vi "Test Cases - API String Arguments Support(VIM).vi"() -> ()   [LabVIEW 2017]
uses:
  2cad2108-17ff-40c4-9c59-29e42dc34fa8.vi
  231c1589-fa39-469a-ad8c-c9d32191fb4b.vi
  479a6c8c-1bad-4955-8cb5-323525784106.vi
  765d0006-b549-469b-b212-20061b8f9c1c.vi
  f8b4bf0f-4264-4187-acce-03e1cac2871a.vi
  390a4868-a891-46e3-9b2d-5b6d63a8fc62.vi
  999417b7-6b4c-4b35-b299-f97fc88c48ae.vi
  e19d2a81-0814-4900-868e-35c1a41a190a.vi
  f192a86a-4283-420b-8c99-03ad7a20a184.vi
  e1086961-258c-488b-92a6-4c27b59b2923.vi
  68628d2e-6ea5-433a-a027-c32794422804.vi
  23749281-1039-457a-b950-e2c2784c1fed.vi
  79993085-fdde-4ff4-95ba-e023c3552d6a.vi
  API-String-Arugments-Support/_Support/Convert API String Arguments to Data(variant).vi
panel:
  out "Cluster":cluster{"2d":dbl[][]}={"2d"=[[3.12, 4.113, 2.3, 5.0, 5.0, 2.3, 4.11, 5.0]]}
  in  "String 13":string="[3.12,4.113,2.3,5;3.12,5,2.3;3.12,4.11,5]"
  out "error 13":errorcluster
  in  "String 12":string="[3.12,4.113,2.3,5;3.12,5,2.3;3.12,4.11,5]"
  out "error 12":errorcluster
  out "Data 11":dbl[][](array[numeric])=[[3.12, 4.113, 2.3, 5.0, 5.0, 2.3, 4.11, 5.0]]
  in  "String 11":string="[{Bool:Off;child.name:ddd},{Bool:On;name:ddd}]"
  out "error 11":errorcluster
  out "Data 10":T1(array[cluster])=[{"Name"="", "Child"={"Name"="ddd"}, "Bool"=FALSE}, {"Name"="ddd", "Child"={"Name"=""}, "Bool"=TRUE}]
  in  "String 10":string="C:\\ni-rt\\data\\a\\2023.07.25"
  out "error 10":errorcluster
  out "Data 9":path=path "C:/ni-rt/data/a/2023.07.25"
  in  "String 9":string="Bool:Off;child.name:ddd"
  out "error 9":errorcluster
  out "Data 8":T2={"Name"="abc", "Child"={"Name"="ddd"}, "Bool"=FALSE}
  in  "String 8":string="[3.12,4.11,5]"
  out "error 8":errorcluster
  out "Data 4":dbl[](array[numeric])=[3.12, 4.11, 5.0]
  in  "String 7":string="ccccc"
  out "error 7":errorcluster
  out "Data 7":enum16{"1 - aaaa", "2 - bbbb", "555 - ccccc"}(ring)=enum."555 - ccccc"
  in  "String 6":string="555"
  out "error 6":errorcluster
  out "Data 6":enum16{"1 - aaaa", "2 - bbbb", "555 - ccccc"}(ring)=enum."555 - ccccc"
  in  "String 5":string="bbbb"
  out "error 5":errorcluster
  out "Data 5":enum16{"aaaa", "bbbb", "ccccc"}(ring)=enum."bbbb"
  in  "String 4":string="3.1415926"
  out "error 4":errorcluster
  out "Data 4":dbl=3.1415926
  in  "String 3":string="0x42"
  out "error 3":errorcluster
  out "Data 3":i32=66
  in  "String 2":string="Enable"
  out "error 2":errorcluster
  out "Data 2":bool=TRUE
  out "Data 1":string="abcd"
  out "error 1":errorcluster
  in  "String":string="abcd"
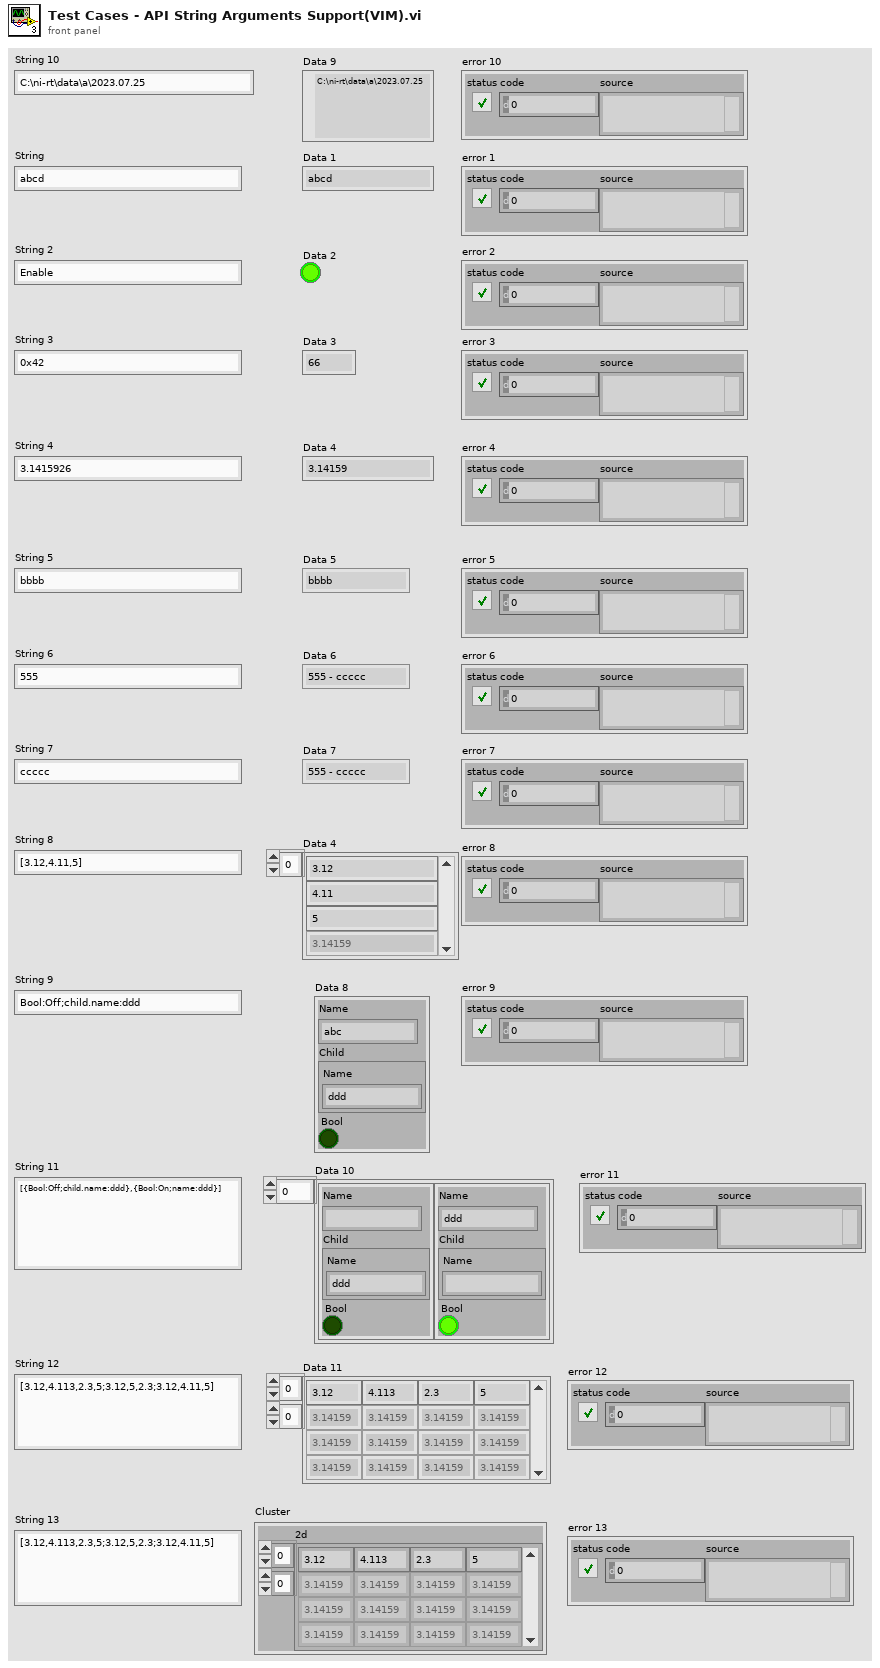
[diagram p1: front panel]
types:
  T1 = cluster{"Name":string, "Child":cluster{"Name":string}, "Bool":bool}[]
  T2 = cluster{"Name":string, "Child":cluster{"Name":string}, "Bool":bool}
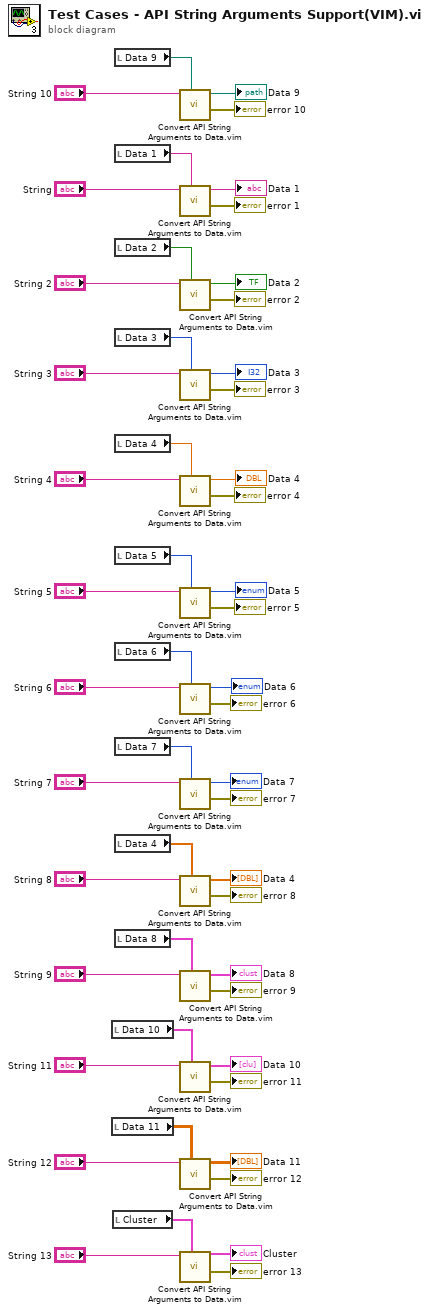
[diagram p0: block diagram]
diagram:
  n1 = local read "Data 10"() -> (w9:T1)
  n2 = local read "Data 11"() -> (w5:dbl[][])
  n3 = local read "Cluster"() -> (w1:cluster{"2d":dbl[][]})
  n4 = local read "Data 9"() -> (w13:path)
  n5 = local read "Data 1"() -> (w52:string)
  n6 = local read "Data 2"() -> (w51:bool)
  n7 = local read "Data 3"() -> (w50:i32)
  n8 = local read "Data 4"() -> (w49:dbl)
  n9 = local read "Data 5"() -> (w48:enum16{"aaaa", "bbbb", "ccccc"})
  n10 = local read "Data 6"() -> (w47:enum16{"1 - aaaa", "2 - bbbb", "555 - ccccc"})
  n11 = local read "Data 7"() -> (w46:enum16{"1 - aaaa", "2 - bbbb", "555 - ccccc"})
  n12 = local read "Data 4"() -> (w45:dbl[])
  n13 = local read "Data 8"() -> (w44:T2)
  n14 = call "Convert API String Arguments to Data.vim"("Type"=w13, "String"="String 10") -> ("error"=→"error 10":errorcluster, "Data"=→"Data 9":path)  [unwired: 6 in]
  n15 = call "Convert API String Arguments to Data.vim"("Type"=w52, "String"="String") -> ("error"=→"error 1":errorcluster, "Data"=→"Data 1":string)  [unwired: 6 in]
  n16 = call "Convert API String Arguments to Data.vim"("Type"=w51, "String"="String 2") -> ("error"=→"error 2":errorcluster, "Data"=→"Data 2":bool)  [unwired: 6 in]
  n17 = call "Convert API String Arguments to Data.vim"("Type"=w50, "String"="String 3") -> ("error"=→"error 3":errorcluster, "Data"=→"Data 3":i32)  [unwired: 6 in]
  n18 = call "Convert API String Arguments to Data.vim"("Type"=w49, "String"="String 4") -> ("error"=→"error 4":errorcluster, "Data"=→"Data 4":dbl)  [unwired: 6 in]
  n19 = call "Convert API String Arguments to Data.vim"("Type"=w48, "String"="String 5") -> ("error"=→"error 5":errorcluster, "Data"=→"Data 5":enum16{"aaaa", "bbbb", "ccccc"})  [unwired: 6 in]
  n20 = call "Convert API String Arguments to Data.vim"("Type"=w47, "String"="String 6") -> ("error"=→"error 6":errorcluster, "Data"=→"Data 6":enum16{"1 - aaaa", "2 - bbbb", "555 - ccccc"})  [unwired: 6 in]
  n21 = call "Convert API String Arguments to Data.vim"("Type"=w46, "String"="String 7") -> ("error"=→"error 7":errorcluster, "Data"=→"Data 7":enum16{"1 - aaaa", "2 - bbbb", "555 - ccccc"})  [unwired: 6 in]
  n22 = call "Convert API String Arguments to Data.vim"("Type"=w45, "String"="String 8") -> ("error"=→"error 8":errorcluster, "Data"=→"Data 4":dbl[])  [unwired: 6 in]
  n23 = call "Convert API String Arguments to Data.vim"("Type"=w44, "String"="String 9") -> ("error"=→"error 9":errorcluster, "Data"=→"Data 8":T2)  [unwired: 6 in]
  n24 = call "Convert API String Arguments to Data.vim"("Type"=w9, "String"="String 11") -> ("error"=→"error 11":errorcluster, "Data"=→"Data 10":T1)  [unwired: 6 in]
  n25 = call "Convert API String Arguments to Data.vim"("Type"=w5, "String"="String 12") -> ("error"=→"error 12":errorcluster, "Data"=→"Data 11":dbl[][])  [unwired: 6 in]
  n26 = call "Convert API String Arguments to Data.vim"("Type"=w1, "String"="String 13") -> ("error"=→"error 13":errorcluster, "Data"=→"Cluster":cluster{"2d":dbl[][]})  [unwired: 6 in]
